vi "Part 2.vi"(11 "Input":string) -> (3 "Output":i64)   [LabVIEW 2021]
uses:
  <userlib>/_OpenG.lib/string/string.llb/Convert EOLs (String)__ogtk.vi
  <vilib>/Analysis/NI_AALPro.lvlib
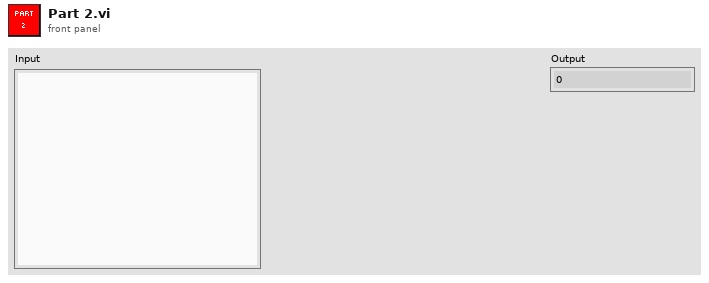
[diagram p1: front panel]
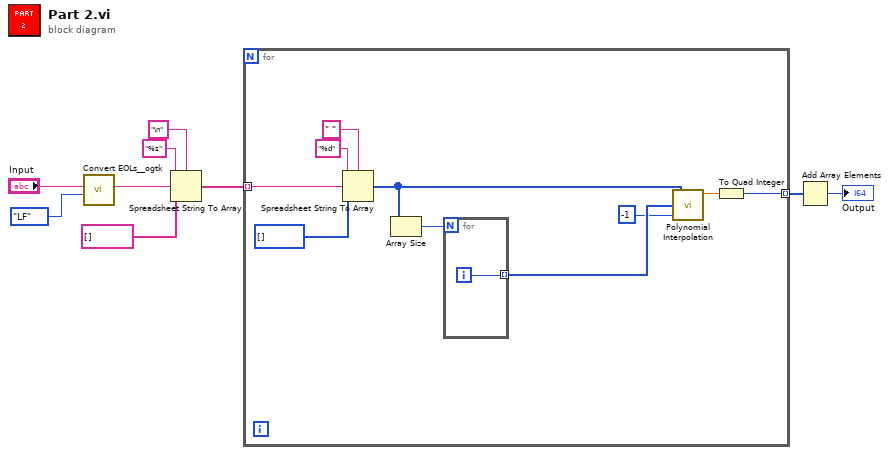
[diagram p0: block diagram]
diagram:
  n1 = call-poly <userlib>:"Convert EOLs__ogtk.vi"("Convert to:"=enum16{"CR", "LF", "CRLF"}."LF", "String in"="Input") -> ("String out"=w5:string)  [unwired: 9 in]
  n2 = Spreadsheet String To Array(delimiter (Tab)="\n", format string="%s", spreadsheet string=w5, array type (2D Dbl)=string[] []) -> (array=w3:string[])
  n3 = for {
    tunnel: w3 -> [w16] mode=indexing
    tunnel: [w11] -> w2 mode=indexing
    n4 = Spreadsheet String To Array(delimiter (Tab)=" ", format string="%d", spreadsheet string=w16, array type (2D Dbl)=i32[] []) -> (array=w14:i32[])
    n5 = Array Size(array=w14) -> (size(s)=w13:i32)
    n6 = for {
      N: w13 -> [_]
      tunnel: [w20] -> w15 mode=indexing
      i -> [w20]
    }
    n7 = call <vilib>:"Polynomial Interpolation.vi"("x value"=-1, "X"=w15, "Y"=w14) -> ("interpolation value"=w12:dbl)  [unwired: 2 out]
    n8 = To Quad Integer(1:w12) -> (0:w11:i64)
  }
  n9 = Add Array Elements(numeric array=w2) -> (sum=→"Output":i64)
